vi "zad2.vi"() -> ()   [LabVIEW 2017]
panel:
  out "Dziesiêtna":dbl
  in  "Dwójkowo":bool[](array[boolean])
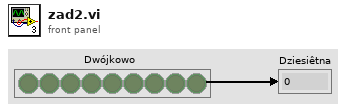
[diagram p1: front panel]
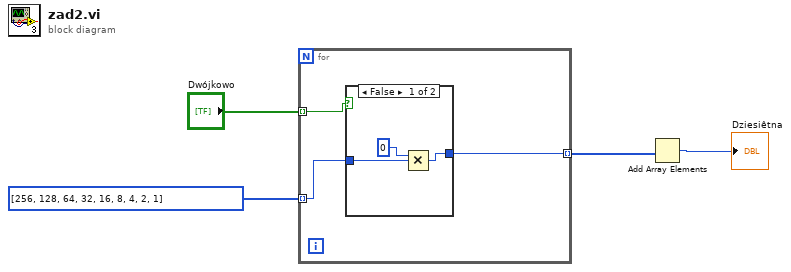
[diagram p0: block diagram]
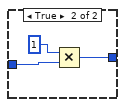
[diagram p2: hidden frame]
diagram:
  n1 = for {
    tunnel: "Dwójkowo" -> [w7] mode=indexing
    tunnel: i32[] [256, 128, 64, 32, 16, 8, 4, 2, 1] -> [w6] mode=indexing
    tunnel: [w5] -> w2 mode=indexing
    n2 = case shown="False" w7 {
      tunnel: w6 -> [w9 w13]
      tunnel: [w8 w11] -> w5
      frame False {
        n3 = Multiply(x=0, y=w9) -> (x*y=w8:i32)
      }
      frame True {
        n4 = Multiply(x=1, y=w13) -> (x*y=w11:i32)
      }
    }
  }
  n5 = Add Array Elements(numeric array=w2) -> (sum=→"Dziesiêtna":i32)
